vi "Func-엑셀 데이터를 그래프로 출력.vi"() -> ()   [LabVIEW 2015] (continued)
25\t34.187\n25\t25\t34.182\n25\t25\t34.179\n25\t25\t34.171\n25\t25\t34.165\n25\t25\t34.161\n25\t25\t34.159\n25\t25\t34.159\n25\t25\t34.161\n25\t25\t34.161\n25\t25\t34.16\n25\t25\t34.159\n25\t25\t34.155\n25\t25\t34.157\n25\t25\t34.155\n25\t25\t34.156\n25\t25\t34.153\n25\t25\t34.152\n25\t25\t34.15\n25\t25\t34.143\n25\t25\t34.141\n25\t25\t34.136\n25\t25\t34.137\n25\t25\t34.134\n25\t25\t34.13\n25\t25\t34.132\n25\t25\t34.132\n25\t25\t34.129\n25\t25\t34.123\n25\t25\t34.123\n25\t25\t34.124\n25\t25\t34.118\n25\t25\t34.111\n25\t25\t34.11\n25\t25\t34.114\n25\t25\t34.11\n25\t25\t34.105\n25\t25\t34.109\n25\t25\t34.106\n25\t25\t34.102\n25\t25\t34.096\n25\t25\t34.093\n25\t25\t34.095\n25\t25\t34.091\n25\t25\t34.093\n25\t25\t34.093\n25\t25\t34.091\n25\t25\t34.085\n25\t25\t34.079\n25\t25\t34.077\n25\t25\t34.071\n25\t25\t34.067\n25\t25\t34.069\n25\t25\t34.071\n25\t25\t34.072\n25\t25\t34.071\n25\t25\t34.068\n25\t25\t34.069\n25\t25\t34.064\n25\t25\t34.065\n25\t25\t34.067\n25\t25\t34.065\n25\t25\t34.063\n25\t25\t34.061\n25\t25\t34.057\n25\t25\t34.054\n25\t25\t34.049\n25\t25\t34.043\n25\t25\t34.044\n25\t25\t34.045\n25\t25\t34.043\n25\t25\t34.041\n25\t25\t34.041\n25\t25\t34.041\n25\t25\t34.034\n25\t25\t34.031\n25\t25\t34.032\n25\t25\t34.031\n25\t25\t34.03\n25\t25\t34.029\n25\t25\t34.029\n25\t25\t34.026\n25\t25\t34.021\n25\t25\t34.02\n25\t25\t34.017\n25\t25\t34.016\n25\t25\t34.017\n25\t25\t34.018\n25\t25\t34.014\n25\t25\t34.01\n25\t25\t34.007\n25\t25\t34.002\n25\t25\t34\n25\t25\t33.997\n25\t25\t33.993\n25\t25\t33.994\n25\t25\t33.996\n25\t25\t33.995\n25\t25\t33.992\n25\t25\t33.992\n25\t25\t33.989\n25\t25\t33.984\n25\t25\t33.979\n25\t25\t33.977\n25\t25\t33.979\n25\t25\t33.974\n25\t25\t33.975\n25\t25\t33.975\n25\t25\t33.975\n25\t25\t33.974\n25\t25\t33.97\n25\t25\t33.967\n25\t25\t33.965\n25\t25\t33.961\n25\t25\t33.954\n25\t25\t33.951\n25\t25\t33.948\n25\t25\t33.946\n25\t25\t33.948\n25\t25\t33.95\n25\t25\t33.949\n25\t25\t33.95\n25\t25\t33.951\n25\t25\t33.949\n25\t25\t33.946\n25\t25\t33.943\n25\t25\t33.945\n25\t25\t33.939\n25\t25\t33.932\n25\t25\t33.928\n25\t25\t33.925\n25\t25\t33.918\n25\t25\t33.914\n25\t25\t33.917\n25\t25\t33.916\n25\t25\t33.914\n25\t25\t33.916\n25\t25\t33.916\n25\t25\t33.916\n25\t25\t33.914\n25\t25\t33.915\n25\t25\t33.917\n25\t25\t33.912\n25\t25\t33.912\n25\t25\t33.91\n25\t25\t33.906\n25\t25\t33.903\n25\t25\t33.9\n25\t25\t33.902\n25\t25\t33.896\n25\t25\t33.896\n25\t25\t33.896\n25\t25\t33.896\n25\t25\t33.895\n25\t25\t33.889\n25\t25\t33.888\n25\t25\t33.885\n25\t25\t33.884\n25\t25\t33.88\n25\t25\t33.878\n25\t25\t33.876\n25\t25\t33.875\n25\t25\t33.875\n25\t25\t33.873\n25\t25\t33.871\n25\t25\t33.869\n25\t25\t33.869\n25\t25\t33.868\n25\t25\t33.865\n25\t25\t33.861\n25\t25\t33.859\n25\t25\t33.859\n25\t25\t33.858\n25\t25\t33.856\n25\t25\t33.856\n25\t25\t33.851\n25\t25\t33.85\n25\t25\t33.846\n25\t25\t33.845\n25\t25\t33.845\n25\t25\t33.842\n25\t25\t33.841\n25\t25\t33.838\n25\t25\t33.839\n25\t25\t33.836\n25\t25\t33.832\n25\t25\t33.83\n25\t25\t33.829\n25\t25\t33.827\n25\t25\t33.826\n25\t25\t33.824\n25\t25\t33.823\n25\t25\t33.821\n25\t25\t33.82\n25\t25\t33.82\n25\t25\t33.822\n25\t25\t33.821\n25\t25\t33.822\n25\t25\t33.825\n25\t25\t33.821\n25\t25\t33.818\n25\t25\t33.813\n25\t25\t33.813\n25\t25\t33.809\n25\t25\t33.801\n25\t25\t33.799\n25\t25\t33.8\n25\t25\t33.796\n25\t25\t33.793\n25\t25\t33.793\n25\t25\t33.789\n25\t25\t33.787\n25\t25\t33.787\n25\t25\t33.787\n25\t25\t33.784\n25\t25\t33.783\n25\t25\t33.786\n25\t25\t33.787\n25\t25\t33.782\n25\t25\t33.777\n25\t25\t33.777\n25\t25\t33.776\n25\t25\t33.772\n25\t25\t33.77\n25\t25\t33.771\n25\t25\t33.77\n25\t25\t33.768\n25\t25\t33.768\n25\t25\t33.766\n25\t25\t33.763\n25\t25\t33.766\n25\t25\t33.764\n25\t25\t33.764\n25\t25\t33.761\n25\t25\t33.757\n25\t25\t33.757\n25\t25\t33.751\n25\t25\t33.749\n25\t25\t33.746\n25\t25\t33.741\n25\t25\t33.74\n25\t25\t33.739\n25\t25\t33.737\n25\t25\t33.734\n25\t25\t33.736\n25\t25\t33.74\n25\t25\t33.741\n25\t25\t33.737\n25\t25\t33.735\n25\t25\t33.734\n25\t25\t33.733\n25\t25\t33.73\n25\t25\t33.727\n25\t25\t33.73\n25\t25\t33.731\n25\t25\t33.731\n25\t25\t33.732\n25\t25\t33.728\n25\t25\t33.726\n25\t25\t33.721\n25\t25\t33.721\n25\t25\t33.718\n25\t25\t33.714\n25\t25\t33.715\n25\t25\t33.714\n25\t25\t33.711\n25\t25\t33.702\n25\t25\t33.705\n25\t25\t33.698\n25\t25\t33.698\n25\t25\t33.697\n25\t25\t33.699\n25\t25\t33.702\n25\t25\t33.697\n25\t25\t33.696\n25\t25\t33.692\n25\t25\t33.69\n25\t25\t33.687\n25\t25\t33.684\n25\t25\t33.681\n25\t25\t33.684\n25\t25\t33.687\n25\t25\t33.687\n25\t25\t33.683\n25\t25\t33.682\n25\t25\t33.679\n25\t25\t33.676\n25\t25\t33.673\n25\t25\t33.671\n25\t25\t33.67\n25\t25\t33.67\n25\t25\t33.673\n25\t25\t33.667\n25\t25\t33.666\n25\t25\t33.664\n25\t25\t33.661\n25\t25\t33.661\n25\t25\t33.659\n25\t25\t33.657\n25\t25\t33.654\n25\t25\t33.652\n25\t25\t33.653\n25\t25\t33.654\n25\t25\t33.649\n25\t25\t33.647\n25\t25\t33.645\n25\t25\t33.644\n25\t25\t33.643\n25\t25\t33.636\n25\t25\t33.637\n25\t25\t33.638\n25\t25\t33.635\n25\t25\t33.631\n25\t25\t33.627\n25\t25\t33.628\n25\t25\t33.625\n25\t25\t33.623\n25\t25\t33.626\n25\t25\t33.627\n25\t25\t33.627\n25\t25\t33.626\n25\t25\t33.623\n25\t25\t33.62\n25\t25\t33.619\n25\t25\t33.62\n25\t25\t33.617\n25\t25\t33.619\n25\t25\t33.616\n25\t25\t33.618\n25\t25\t33.616\n25\t25\t33.612\n25\t25\t33.611\n25\t25\t33.605\n25\t25\t33.607\n25\t25\t33.602\n25\t25\t33.601\n25\t25\t33.6\n25\t25\t33.598\n25\t25\t33.598\n25\t25\t33.598\n25\t25\t33.6\n25\t25\t33.596\n25\t25\t33.596\n25\t25\t33.593\n25\t25\t33.594\n25\t25\t33.595\n25\t25\t33.591\n25\t25\t33.589\n25\t25\t33.586\n25\t25\t33.589\n25\t25\t33.587\n25\t25\t33.579\n25\t25\t33.58\n25\t25\t33.579\n25\t25\t33.582\n25\t25\t33.579\n25\t25\t33.577\n25\t25\t33.575\n25\t25\t33.575\n25\t25\t33.571\n25\t25\t33.565\n25\t25\t33.567\n25\t25\t33.567\n25\t25\t33.571\n25\t25\t33.566\n25\t25\t33.57\n25\t25\t33.568\n25\t25\t33.565\n25\t25\t33.559\n25\t25\t33.555\n25\t25\t33.554\n25\t25\t33.547\n25\t25\t33.549\n25\t25\t33.549\n25\t25\t33.555\n25\t25\t33.555\n25\t25\t33.557\n25\t25\t33.557\n25\t25\t33.554\n25\t25\t33.552\n25\t25\t33.548\n25\t25\t33.544\n25\t25\t33.541\n25\t25\t33.537\n25\t25\t33.533\n25\t25\t33.528\n25\t25\t33.527\n25\t25\t33.532\n25\t25\t33.532\n25\t25\t33.532\n25\t25\t33.534\n25\t25\t33.532\n25\t25\t33.53\n25\t25\t33.526\n25\t25\t33.524\n25\t25\t33.526\n25\t25\t33.527\n25\t25\t33.524\n25\t25\t33.521\n25\t25\t33.519\n25\t25\t33.518\n25\t25\t33.512\n25\t25\t33.509\n25\t25\t33.512\n25\t25\t33.512\n25\t25\t33.513\n25\t25\t33.509\n25\t25\t33.513\n25\t25\t33.513\n25\t25\t33.512\n25\t25\t33.511\n25\t25\t33.508\n25\t25\t33.508\n25\t25\t33.506\n25\t25\t33.501\n25\t25\t33.5\n25\t25\t33.498\n25\t25\t33.496\n25\t25\t33.496\n25\t25\t33.493\n25\t25\t33.494\n25\t25\t33.49\n25\t25\t33.487\n25\t25\t33.486\n25\t25\t33.486\n25\t25\t33.486\n25\t25\t33.484\n25\t25\t33.482\n25\t25\t33.483\n25\t25\t33.486\n25\t25\t33.483\n25\t25\t33.482\n25\t25\t33.478\n25\t25\t33.481\n25\t25\t33.482\n25\t25\t33.477\n25\t25\t33.474\n25\t25\t33.476\n25\t25\t33.476\n25\t25\t33.471\n25\t25\t33.468\n25\t25\t33.465\n25\t25\t33.466\n25\t25\t33.465\n25\t25\t33.463\n25\t25\t33.463\n25\t25\t33.461\n25\t25\t33.461\n25\t25\t33.46\n25\t25\t33.457\n25\t25\t33.458\n25\t25\t33.457\n25\t25\t33.459\n25\t25\t33.457\n25\t25\t33.458\n25\t25\t33.454\n25\t25\t33.452\n25\t25\t33.457\n25\t25\t33.453\n25\t25\t33.448\n25\t25\t33.446\n25\t25\t33.45\n25\t25\t33.448\n25\t25\t33.439\n25\t25\t33.44\n25\t25\t33.442\n25\t25\t33.439\n25\t25\t33.437\n25\t25\t33.436\n25\t25\t33.436\n25\t25\t33.433\n25\t25\t33.432\n25\t25\t33.436\n25\t25\t33.43\n25\t25\t33.43\n25\t25\t33.428\n25\t25\t33.426\n25\t25\t33.426\n25\t25\t33.425\n25\t25\t33.424\n25\t25\t33.423\n25\t25\t33.423\n25\t25\t33.424\n25\t25\t33.423\n25\t25\t33.421\n25\t25\t33.423\n25\t25\t33.419\n25\t25\t33.414\n25\t25\t33.415\n25\t25\t33.414\n25\t25\t33.416\n25\t25\t33.411\n25\t25\t33.412\n25\t25\t33.412\n25\t25\t33.409\n25\t25\t33.406\n25\t25\t33.397\n25\t25\t33.402\n25\t25\t33.402\n25\t25\t33.404\n25\t25\t33.406\n25\t25\t33.408\n25\t25\t33.408\n25\t25\t33.405\n25\t25\t33.4\n25\t25\t33.398\n25\t25\t33.393\n25\t25\t33.391\n25\t25\t33.389\n25\t25\t33.385\n25\t25\t33.386\n25\t25\t33.388\n25\t25\t33.389\n25\t25\t33.387\n25\t25\t33.385\n25\t25\t33.388\n25\t25\t33.384\n25\t25\t33.38\n25\t25\t33.378\n25\t25\t33.377\n25\t25\t33.375\n25\t25\t33.37\n25\t25\t33.367\n25\t25\t33.366\n25\t25\t33.368\n25\t25\t33.364\n25\t25\t33.362\n25\t25\t33.361\n25\t25\t33.362\n25\t25\t33.362\n25\t25\t33.359\n25\t25\t33.362\n25\t25\t33.363\n25\t25\t33.36\n25\t25\t33.357\n25\t25\t33.355\n25\t25\t33.354\n25\t25\t33.351\n25\t25\t33.348\n25\t25\t33.353\n25\t25\t33.357\n25\t25\t33.355\n25\t25\t33.355\n25\t25\t33.354\n25\t25\t33.355\n25\t25\t33.355\n25\t25\t33.349\n25\t25\t33.348\n25\t25\t33.349\n25\t25\t33.349\n25\t25\t33.349\n25\t25\t33.346\n25\t25\t33.349\n25\t25\t33.347\n25\t25\t33.345\n25\t25\t33.342\n25\t25\t33.339\n25\t25\t33.336\n25\t25\t33.331\n25\t25\t33.332\n25\t25\t33.332\n25\t25\t33.33\n25\t25\t33.328\n25\t25\t33.328\n25\t25\t33.33\n25\t25\t33.328\n25\t25\t33.326\n25\t25\t33.327\n25\t25\t33.33\n25\t25\t33.327\n25\t25\t33.325\n25\t25\t33.327\n25\t25\t33.321\n25\t25\t33.321\n25\t25\t33.317\n25\t25\t33.313\n25\t25\t33.312\n25\t25\t33.309\n25\t25\t33.312\n25\t25\t33.308\n25\t25\t33.306\n25\t25\t33.306\n25\t25\t33.306\n25\t25\t33.307\n25\t25\t33.307\n25\t25\t33.306\n25\t25\t33.307\n25\t25\t33.306\n25\t25\t33.303\n25\t25\t33.303\n25\t25\t33.3\n25\t25\t33.302\n25\t25\t33.304\n25\t25\t33.306\n25\t25\t33.305\n25\t25\t33.3\n25\t25\t33.297\n25\t25\t33.295\n25\t25\t33.291\n25\t25\t33.285\n25\t25\t33.287\n25\t25\t33.287\n25\t25\t33.289\n25\t25\t33.287\n25\t25\t33.285\n25\t25\t33.287\n25\t25\t33.281\n25\t25\t33.282\n25\t25\t33.279\n25\t25\t33.278\n25\t25\t33.277\n25\t25\t33.28\n25\t25\t33.281\n25\t25\t33.28\n25\t25\t33.276\n25\t25\t33.275\n25\t25\t33.276\n25\t25\t33.274\n25\t25\t33.275\n25\t25\t33.272\n25\t25\t33.275\n25\t25\t33.277\n25\t25\t33.276\n25\t25\t33.273\n25\t25\t33.27\n25\t25\t33.268\n25\t25\t33.264\n25\t25\t33.259\n25\t25\t33.256\n25\t25\t33.257\n25\t25\t33.258\n25\t25\t33.256\n25\t25\t33.257\n25\t25\t33.257\n25\t25\t33.255\n25\t25\t33.257\n25\t25\t33.258\n25\t25\t33.26\n25\t25\t33.259\n25\t25\t33.26\n25\t25\t33.262\n25\t25\t33.257\n25\t25\t33.254\n25\t25\t33.254\n25\t25\t33.254\n25\t25\t33.254\n25\t25\t33.252\n25\t25\t33.25\n25\t25\t33.247\n25\t25\t33.246\n25\t25\t33.246\n25\t25\t33.243\n25\t25\t33.239\n25\t25\t33.238\n25\t25\t33.24\n25\t25\t33.238\n25\t25\t33.236\n25\t25\t33.233\n25\t25\t33.236\n25\t25\t33.238\n25\t25\t33.238\n25\t25\t33.239\n25\t25\t33.239\n25\t25\t33.237\n25\t25\t33.233\n25\t25\t33.23\n25\t25\t33.225\n25\t25\t33.225\n25\t25\t33.223\n25\t25\t33.229\n25\t25\t33.229\n25\t25\t33.23\n25\t25\t33.229\n25\t25\t33.229\n25\t25\t33.225\n25\t25\t33.223\n25\t25\t33.222\n25\t25\t33.218\n25\t25\t33.221\n25\t25\t33.216\n25\t25\t33.216\n25\t25\t33.213\n25\t25\t33.215\n25\t25\t33.216\n25\t25\t33.21\n25\t25\t33.21\n25\t25\t33.212\n25\t25\t33.211\n25\t25\t33.205\n25\t25\t33.207\n25\t25\t33.209\n25\t25\t33.209\n25\t25\t33.209\n25\t25\t33.207\n25\t25\t33.209\n25\t25\t33.205\n25\t25\t33.207\n25\t25\t33.208\n25\t25\t33.201\n25\t25\t33.198\n25\t25\t33.196\n25\t25\t33.193\n25\t25\t33.192\n25\t25\t33.192\n25\t25\t33.197\n25\t25\t33.199\n25\t25\t33.201\n25\t25\t33.198\n25\t25\t33.196\n25\t25\t33.195\n25\t25\t33.19\n25\t25\t33.193\n25\t25\t33.189\n25\t25\t33.192\n25\t25\t33.192\n25\t25\t33.189\n25\t25\t33.193\n25\t25\t33.191\n25\t25\t33.196\n25\t25\t33.192\n25\t25\t33.192\n25\t25\t33.19\n25\t25\t33.188\n25\t25\t33.188\n25\t25\t33.182\n25\t25\t33.186\n25\t25\t33.183\n25\t25\t33.18\n25\t25\t33.178\n25\t25\t33.176\n25\t25\t33.176\n25\t25\t33.172\n25\t25\t33.172\n25\t25\t33.173\n25\t25\t33.171\n25\t25\t33.168\n25\t25\t33.167\n25\t25\t33.167\n25\t25\t33.167\n25\t25\t33.166\n25\t25\t33.165\n25\t25\t33.165\n25\t25\t33.164\n25\t25\t33.164\n25\t25\t33.161\n25\t25\t33.161\n25\t25\t33.163\n25\t25\t33.163\n25\t25\t33.162\n25\t25\t33.158\n25\t25\t33.155\n25\t25\t33.155\n25\t25\t33.153\n25\t25\t33.152\n25\t25\t33.15\n25\t25\t33.152\n25\t25\t33.156\n25\t25\t33.151\n25\t25\t33.151\n25\t25\t33.15\n25\t25\t33.151\n25\t25\t33.15\n25\t25\t33.148\n25\t25\t33.15\n25\t25\t33.15\n25\t25\t33.15\n25\t25\t33.15\n25\t25\t33.15\n25\t25\t33.148\n25\t25\t33.147\n25\t25\t33.145\n25\t25\t33.147\n25\t25\t33.143\n25\t25\t33.144\n25\t25\t33.146\n25\t25\t33.147\n25\t25\t33.141\n25\t25\t33.141\n25\t25\t33.139\n25\t25\t33.134\n25\t25\t33.131\n25\t25\t33.131\n25\t25\t33.134\n25\t25\t33.132\n25\t25\t33.132\n25\t25\t33.136\n25\t25\t33.134\n25\t25\t33.13\n25\t25\t33.127\n25\t25\t33.123\n25\t25\t33.122\n25\t25\t33.118\n25\t25\t33.117\n25\t25\t33.121\n25\t25\t33.12\n25\t25\t33.124\n25\t25\t33.125\n25\t25\t33.123\n25\t25\t33.123\n25\t25\t33.118\n25\t25\t33.121\n25\t25\t33.117\n25\t25\t33.118\n25\t25\t33.116\n25\t25\t33.119\n25\t25\t33.119\n25\t25\t33.116\n25\t25\t33.112\n25\t25\t33.109\n25\t25\t33.111\n25\t25\t33.109\n25\t25\t33.108\n25\t25\t33.107\n25\t25\t33.11\n25\t25\t33.106\n25\t25\t33.102\n25\t25\t33.102\n25\t25\t33.102\n25\t25\t33.104\n25\t25\t33.102\n25\t25\t33.102\n25\t25\t33.102\n25\t25\t33.101\n25\t25\t33.099\n25\t25\t33.096\n25\t25\t33.095\n25\t25\t33.097\n25\t25\t33.094\n25\t25\t33.091\n25\t25\t33.09\n25\t25\t33.09\n25\t25\t33.093\n25\t25\t33.092\n25\t25\t33.092\n25\t25\t33.091\n25\t25\t33.089\n25\t25\t33.089\n25\t25\t33.084\n25\t25\t33.08\n25\t25\t33.082\n25\t25\t33.084\n25\t25\t33.082\n25\t25\t33.079\n25\t25\t33.079\n25\t25\t33.08\n25\t25\t33.08\n25\t25\t33.079\n25\t25\t33.079\n25\t25\t33.082\n25\t25\t33.082\n25\t25\t33.08\n25\t25\t33.079\n25\t25\t33.077\n25\t25\t33.079\n25\t25\t33.079\n25\t25\t33.081\n25\t25\t33.081\n25\t25\t33.082\n25\t25\t33.082\n25\t25\t33.082\n25\t25\t33.075\n25\t25\t33.075\n25\t25\t33.073\n25\t25\t33.072\n25\t25\t33.068\n25\t25\t33.065\n25\t25\t33.067\n25\t25\t33.062\n25\t25\t33.062\n25\t25\t33.059\n25\t25\t33.062\n25\t25\t33.059\n25\t25\t33.062\n25\t25\t33.067\n25\t25\t33.064\n25\t25\t33.06\n25\t25\t33.054\n25\t25\t33.057\n25\t25\t33.054\n25\t25\t33.049\n25\t25\t33.051\n25\t25\t33.054\n25\t25\t33.057\n25\t25\t33.056\n25\t25\t33.055\n25\t25\t33.054\n25\t25\t33.053\n25\t25\t33.053\n25\t25\t33.053\n25\t25\t33.055\n25\t25\t33.057\n25\t25\t33.058\n25\t25\t33.062\n25\t25\t33.06\n25\t25\t33.055\n25\t25\t33.052\n25\t25\t33.05\n25\t25\t33.047\n25\t25\t33.042\n25\t25\t33.042\n25\t25\t33.042\n25\t25\t33.039\n25\t25\t33.037\n25\t25\t33.039\n25\t25\t33.04\n25\t25\t33.035\n25\t25\t33.035\n25\t25\t33.039\n25\t25\t33.039\n25\t25\t33.036\n25\t25\t33.034\n25\t25\t33.034\n25\t25\t33.036\n25\t25\t33.033\n25\t25\t33.031\n25\t25\t33.029\n25\t25\t33.025\n25\t25\t33.03\n25\t25\t33.026\n25\t25\t33.023\n25\t25\t33.027\n25\t25\t33.03\n25\t25\t33.033\n24.917\t24.94\t32.646\n24.833\t24.87\t32.65\n24.75\t25.01\t32.648\n24.667\t24.98\t32.644\n24.583\t24.95\t32.64\n24.5\t24.89\t32.639\n24.417\t24.84\t32.637\n24.333\t24.78\t32.63\n24.25\t24.71\t32.639\n24.167\t24.64\t32.633\n24.083\t24.57\t32.635\n24\t24.5\t32.632\n23.917\t24.42\t32.628\n23.833\t24.34\t32.621\n23.75\t24.26\t32.626\n23.667\t24.17\t32.61\n23.583\t24.08\t32.622\n23.5\t23.99\t32.625\n23.417\t23.91\t32.617\n23.333\t23.83\t32.606\n23.25\t23.73\t32.604\n23.167\t23.65\t32.606\n23.083\t23.58\t32.595\n23\t23.51\t32.593\n22.917\t23.44\t32.58\n22.833\t23.37\t32.578\n22.75\t23.28\t32.571\n22.667\t23.2\t32.566\n22.583\t23.12\t32.559\n22.5\t23.02\t32.551\n22.417\t22.94\t32.541\n22.333\t22.86\t32.531\n22.25\t22.78\t32.53\n22.167\t22.71\t32.513\n22.083\t22.63\t32.503\n22\t22.56\t32.493\n21.917\t22.48\t32.481\n21.833\t22.37\t32.469\n21.75\t22.18\t32.454\n21.667\t21.89\t32.446\n21.583\t21.54\t32.438\n21.5\t21.12\t32.416\n21.417\t20.64\t32.4\n21.333\t20.14\t32.387\n21.25\t19.64\t32.37\n21.167\t19.15\t32.355\n21.083\t18.72\t32.337\n21\t18.32\t32.318\n20.917\t17.96\t32.283\n20.833\t17.65\t32.26\n20.75\t17.38\t32.245\n20.667\t17.17\t32.215\n20.583\t16.99\t32.19\n20.5\t16.85\t32.154\n20.417\t16.74\t32.12\n20.333\t16.66\t32.085\n20.25\t16.61\t32.057\n20.167\t16.57\t32.018\n20.083\t16.54\t31.975\n20\t16.54\t31.934\n19.917\t16.54\t31.885\n19.833\t16.56\t31.85\n19.75\t16.57\t31.793\n19.667\t16.59\t31.748\n19.583\t16.61\t31.706\n19.5\t16.63\t31.647\n19.417\t16.66\t31.601\n19.333\t16.66\t31.559\n19.25\t16.68\t31.488\n19.167\t16.69\t31.442\n19.083\t16.69\t31.391\n19\t16.7\t31.323\n18.917\t16.68\t31.273\n18.833\t16.66\t31.209\n18.75\t16.65\t31.157\n18.667\t16.62\t31.095\n18.583\t16.58\t31.039\n18.5\t16.56\t30.975\n18.417\t16.51\t30.926\n18.333\t16.48\t30.867\n18.25\t16.42\t30.803\n18.167\t16.36\t30.74\n18.083\t16.3\t30.68\n18\t16.23\t30.621\n17.917\t16.16\t30.561\n17.833\t16.1\t30.507\n17.75\t16.04\t30.448\n17.667\t15.96\t30.384\n17.583\t15.87\t30.312\n17.5\t15.79\t30.263\n17.417\t15.7\t30.192\n17.333\t15.62\t30.129\n17.25\t15.53\t30.076\n17.167\t15.45\t30.013\n17.083\t15.35\t29.941\n17\t15.27\t29.896\n16.917\t15.18\t29.831\n16.833\t15.08\t29.769\n16.75\t14.99\t29.703\n16.667\t14.9\t29.649\n16.583\t14.81\t29.581\n16.5\t14.72\t29.527\n16.417\t14.64\t29.461\n16.333\t14.55\t29.398\n16.25\t14.46\t29.327\n16.167\t14.37\t29.275\n16.083\t14.28\t29.205\n16\t14.2\t29.143\n15.917\t14.13\t29.079\n15.833\t14.04\t29.018\n15.75\t13.95\t28.959\n15.667\t13.87\t28.88\n15.583\t13.79\t28.825\n15.5\t13.71\t28.763\n15.417\t13.63\t28.698\n15.333\t13.54\t28.634\n15.25\t13.46\t28.573\n15.167\t13.38\t28.516\n15.083\t13.3\t28.45\n15\t13.23\t28.388\n14.917\t13.15\t28.325\n14.833\t13.07\t28.247\n14.75\t12.99\t28.181\n14.667\t12.91\t28.118\n14.583\t12.83\t28.054\n14.5\t12.75\t28\n14.417\t12.67\t27.923\n14.333\t12.6\t27.859\n14.25\t12.53\t27.794\n14.167\t12.45\t27.729\n14.083\t12.37\t27.655\n14\t12.28\t27.597\n13.917\t12.21\t27.527\n13.833\t12.11\t27.475\n13.75\t12.04\t27.404\n13.667\t11.97\t27.339\n13.583\t11.89\t27.271\n13.5\t11.8\t27.198\n13.417\t11.71\t27.132\n13.333\t11.64\t27.063\n13.25\t11.55\t26.998\n13.167\t11.46\t26.934\n13.083\t11.37\t26.862\n13\t11.28\t26.794\n12.917\t11.2\t26.726\n12.833\t11.13\t26.663\n12.75\t11.04\t26.589\n12.667\t10.96\t26.523\n12.583\t10.88\t26.456\n12.5\t10.8\t26.394\n12.417\t10.73\t26.316\n12.333\t10.65\t26.251\n12.25\t10.55\t26.181\n12.167\t10.47\t26.106\n12.083\t10.39\t26.044\n12\t10.31\t25.974\n11.917\t10.25\t25.908\n11.833\t10.17\t25.84\n11.75\t10.09\t25.765\n11.667\t10.02\t25.699\n11.583\t9.95\t25.634\n11.5\t9.87\t25.564\n11.417\t9.78\t25.49\n11.333\t9.7\t25.423\n11.25\t9.62\t25.357\n11.167\t9.54\t25.28\n11.083\t9.46\t25.218\n11\t9.38\t25.149\n10.917\t9.3\t25.078\n10.833\t9.22\t25.007\n10.75\t9.14\t24.946\n10.667\t9.07\t24.862\n10.583\t8.99\t24.801\n10.5\t8.9\t24.725\n10.417\t8.82\t24.659\n10.333\t8.73\t24.583\n10.25\t8.66\t24.516\n10.167\t8.58\t24.448\n10.083\t8.5\t24.377\n10\t8.43\t24.299\n9.917\t8.35\t24.227\n9.833\t8.27\t24.162\n9.75\t8.19\t24.096\n9.667\t8.11\t24.014\n9.583\t8.03\t23.954\n9.5\t7.95\t23.886\n9.417\t7.88\t23.814\n9.333\t7.79\t23.747\n9.25\t7.71\t23.672\n9.167\t7.63\t23.6\n9.083\t7.55\t23.53\n9\t7.47\t23.462\n8.917\t7.38\t23.377\n8.833\t7.31\t23.314\n8.75\t7.23\t23.25\n8.667\t7.15\t23.166\n8.583\t7.07\t23.096\n8.5\t6.97\t23.033\n8.417\t6.89\t22.965\n8.333\t6.81\t22.885\n8.25\t6.72\t22.82\n8.167\t6.63\t22.745\n8.083\t6.56\t22.675\n8\t6.48\t22.589\n7.917\t6.4\t22.523\n7.833\t6.32\t22.451\n7.75\t6.24\t22.379\n7.667\t6.16\t22.308\n7.583\t6.07\t22.24\n7.5\t5.99\t22.171\n7.417\t5.91\t22.089\n7.333\t5.82\t22.023\n7.25\t5.74\t21.947\n7.167\t5.67\t21.869\n7.083\t5.59\t21.802\n7\t5.52\t21.729\n6.917\t5.44\t21.652\n6.833\t5.37\t21.584\n6.75\t5.29\t21.518\n6.667\t5.22\t21.444\n6.583\t5.14\t21.37\n6.5\t5.05\t21.292\n6.417\t4.97\t21.222\n6.333\t4.89\t21.145\n6.25\t4.81\t21.075\n6.167\t4.73\t21.011\n6.083\t4.64\t20.932\n6\t4.56\t20.852\n5.917\t4.49\t20.784\n5.833\t4.41\t20.711\n5.75\t4.33\t20.627\n5.667\t4.27\t20.568\n5.583\t4.19\t20.493\n5.5\t4.12\t20.418\n5.417\t4.04\t20.343\n5.333\t3.96\t20.276\n5.25\t3.88\t20.198\n5.167\t3.8\t20.129\n5.083\t3.72\t20.056\n5\t3.64\t19.978\n4.917\t3.55\t19.907\n4.833\t3.47\t19.837\n4.75\t3.4\t19.763\n4.667\t3.32\t19.691\n4.583\t3.23\t19.62\n4.5\t3.15\t19.538\n4.417\t3.07\t19.468\n4.333\t2.99\t19.393\n4.25\t
